vi "VIW Read.vi"(7 "error in":errorcluster, 8 "String command":string, 10 "VISA resource name in":refnum<visa-resource-name>) -> (0 "error out":errorcluster, 1 "Converted":dbl, 2 "Stop":bool, 3 "VISA resource name out":refnum<visa-resource-name>, 4 "FS 2":T1={"A"=2.0, "V"=2.0, "TRI\\MONO"=2.0, "A*10?"=FALSE} {"TRI\\MONO" items=["MONOFASE", "TRIFASE"]})   [LabVIEW 2016]
panel:
  out "element":bool
  out "result":bool
  out "libero1 2":bool
  out "libero1":bool
  out "Check last 2bit(T=OK)":bool
  out "Converted 2":dbl
  out "return count":u32
  out "Bytes at Port":u32
  out "read buffer":string
  out "Serial Settings:Number of Bytes at Serial Port":u32
  # "Deve essere compreso\ntra 1 e 9"
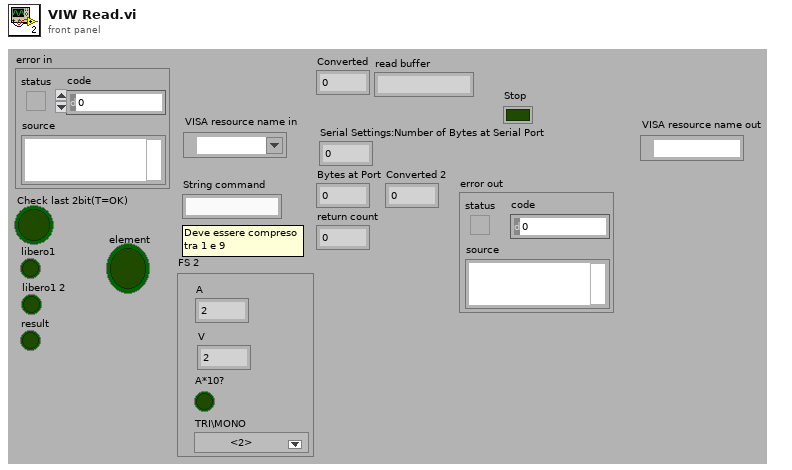
[diagram p1: front panel]
types:
  T1 = cluster{"A":dbl, "V":dbl, "TRI\\MONO":dbl, "A*10?":bool}
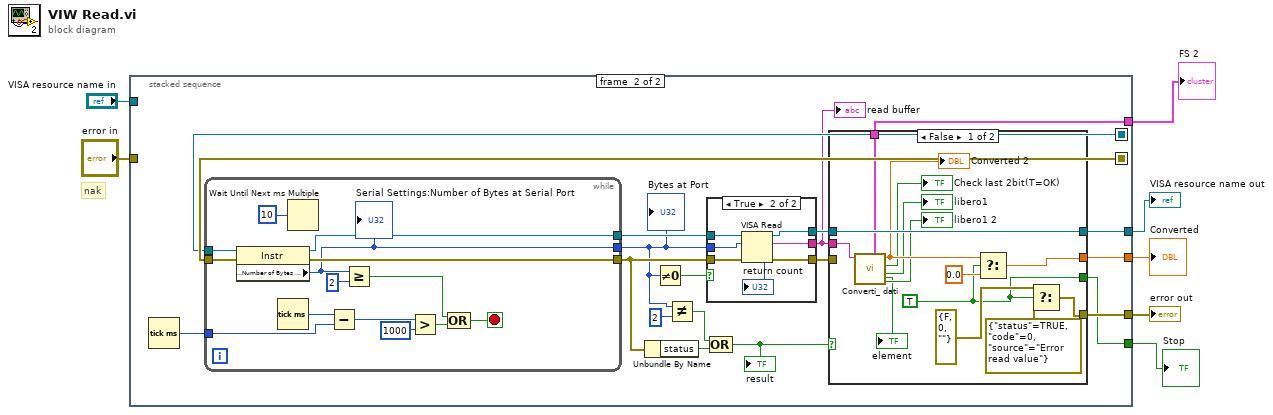
[diagram p0: block diagram]
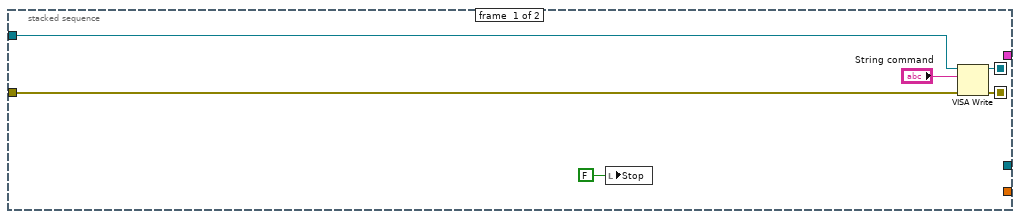
[diagram p2: hidden frame]
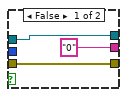
[diagram p3: hidden frame]
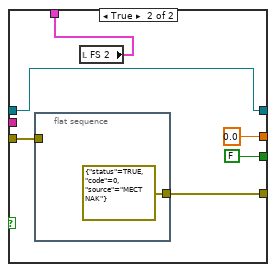
[diagram p4: hidden frame]
diagram:
  # "nak"
  n1 = stacked-sequence {
    seq-local: [w13 _] -> [_ w24]
    seq-local: [w12 _] -> [_ w32]
    tunnel: [_ w26] -> w6
    tunnel: "VISA resource name in" -> [w11 _]
    tunnel: [_ w31] -> w5
    tunnel: "error in" -> [w10 _]
    tunnel: [_ w25] -> w3
    tunnel: [_ w16] -> w2
    tunnel: [_ w14] -> w1
    frame #0 {
      n2 = local write "Stop"(FALSE ("Stop")) -> ()
      n3 = VISA Write(VISA resource name=w11, write buffer="String command", error in (no error)=w10) -> (VISA resource name out=w13:refnum<visa-resource-name>, error out=w12:errorcluster)  [unwired: 1 out]
    }
    frame #1 {
      n4 = Tick Count (ms)() -> (millisecond timer value=w27:u32)
      n5 = while {
        tunnel: w24 -> [w56]
        tunnel: w32 -> [w55]
        tunnel: [w51] -> w21
        tunnel: [w47] -> w18
        tunnel: [w50] -> w22
        tunnel: w27 -> [w44]
        stop <- w45 stop-if-true
        n6 = property class="Instr"(reference=w56, error in=w55) -> (reference out=w50:refnum<visa-resource-name>, error out=w51:errorcluster, "Serial Settings:Number of Bytes at Serial Port"=w47:u32)
        "Serial Settings:Number of Bytes at Serial Port" <- w47
        n7 = Tick Count (ms)() -> (millisecond timer value=w54:u32)
        n8 = Wait Until Next ms Multiple(millisecond multiple=u32 10) -> ()  [unwired: 1 out]
        n9 = Subtract(x=w54, y=w44) -> (x-y=w53:u32)
        n10 = Greater Or Equal?(x=w47, y=2) -> (x >= y?=w46:bool)
        n11 = Greater?(x=w53, y=1000) -> (0:w49:bool)
        n12 = Compound Arithmetic op=OR(w46, w49) -> (w45:bool)
      }
      "Bytes at Port" <- w18
      n13 = Unbundle By Name(w21) -> ("status"=w23:bool)
      n14 = Not Equal To 0?(x=w18) -> (x != 0?=w19:bool)
      n15 = Not Equal?(x=w18, y=2) -> (x != y?=w28:bool)
      n16 = case shown="True" w19 {
        tunnel: w22 -> [w35 w42]
        tunnel: w21 -> [w34 w41]
        tunnel: [w35 w40] -> w20
        tunnel: [w34 w39] -> w15
        tunnel: w18 -> [_ w38]
        tunnel: ["0" ("read buffer") w37] -> w17
        frame False {
        }
        frame True {
          n17 = VISA Read(VISA resource name=w42, byte count=w38, error in (no error)=w41) -> (VISA resource name out=w40:refnum<visa-resource-name>, read buffer=w37:string, return count=→"return count":u32, error out=w39:errorcluster)
        }
      }
      "read buffer" <- w17
      n18 = Compound Arithmetic op=OR(w28, w23) -> (w30:bool)
      "result" <- w30
      n19 = case shown="False" w30 {
        tunnel: [w64 w76] -> w26
        tunnel: [w70 w74] -> w31
        tunnel: w20 -> [w70 w74]
        tunnel: w15 -> [_ w73]
        tunnel: [w68 0.0 ("Converted")] -> w25
        tunnel: w17 -> [w69 _]
        tunnel: [w62 FALSE ("Check last 2bit(T=OK)")] -> w16
        tunnel: [w57 w71] -> w14
        frame False {
          w62 = TRUE ("s")
          n20 = call "Converti_ dati.vi"("String in"=w69) -> ("libero1 2"=→"libero1 2":bool, "libero1"=→"libero1":bool, "Check last 2bit(T=OK)"=→"Check last 2bit(T=OK)":bool, "Converted"=w66:dbl, "element"=→"element":bool, "FS 2"=w57:T1)  [unwired: 5 out]
          "Converted 2" <- w66
          n21 = Select(t=w66, s=w62, f=0.0) -> (s? t:f=w68:dbl)
          n22 = Select(t=errorcluster {"status"=FALSE, "code"=0, "source"=""} ("error out 2"), s=w62, f=errorcluster {"status"=TRUE, "code"=0, "source"="Error read value"} ("error out 2")) -> (s? t:f=w64:errorcluster)
        }
        frame True {
          n23 = flat-sequence {
            tunnel: [errorcluster {"status"=TRUE, "code"=0, "source"="MECT NAK"} ("error out 2")] -> w76
            tunnel: w73 -> [_]
            frame #0 {
            }
          }
          n24 = local read "FS 2"() -> (w71:T1)
        }
      }
    }
  }
  "error out" <- w6
  "VISA resource name out" <- w5
  "Converted" <- w3
  "Stop" <- w2
  "FS 2" <- w1
